vi "Configure Gamepad.vi"(6 "Cluster":T2, 7 "Configuration":T1, 8 "Slide 2":refnum<vi>, 9 "invert y":refnum<vi>, 10 "invert x":refnum<vi>, 11 "device ID":refnum<k1>) -> (3 "Configuration":T1)   [LabVIEW 2012]
uses:
  <vilib>/Utility/miscctls.llb/LVPointTypeDef.ctl
  <vilib>/Utility/inputDevices.llb/joystickAcquire.vi
  <vilib>/Utility/file.llb/Write To Spreadsheet File (I64).vi
  <vilib>/Utility/file.llb/Read From Spreadsheet File (I64).vi
panel:
  out "down":u16(ring) items=["X+", "X-", "Y+", "Y-"]
  out "left":u16(ring) items=["X+", "X-", "Y+", "Y-"]
  in  "right":u16(ring) items=["X+", "X-", "Y+", "Y-"]
  out "V":i32
  out "U":i32
  out "Left Y":i32
  out "B":i32
  out "A":i32
  out "Left X":i32
  out "Right Y":i32
  out "Right X":i32
  in  "close_button":bool
  in  "up":u16(ring) items=["X+", "X-", "Y+", "Y-"]
  in  "load":bool
  in  "save":bool
  in  "Invert":bool
  in  "Invert":bool=TRUE
  in  "Slide":cluster{u32, u32}(slide)={7, 2} scale=0.0..7.0
  out "Settings Refrences":T2
  in  "xr":u16(ring)=1 items=["1 X"=1, "2 A"=2, "3 B"=3, "4 Y"=4, "5 LB"=5, "6 RB"=6, "7 LT"=7, "8 RT"=8, "9 Back"=9]
  in  "yf":u16(ring)=4 items=["1 X"=1, "2 A"=2, "3 B"=3, "4 Y"=4, "5 LB"=5, "6 RB"=6, "7 LT"=7, "8 RT"=8, "9 Back"=9]
  in  "yr":u16(ring)=2 items=["1 X"=1, "2 A"=2, "3 B"=3, "4 Y"=4, "5 LB"=5, "6 RB"=6, "7 LT"=7, "8 RT"=8, "9 Back"=9]
  in  "xf":u16(ring)=3 items=["1 X"=1, "2 A"=2, "3 B"=3, "4 Y"=4, "5 LB"=5, "6 RB"=6, "7 LT"=7, "8 RT"=8, "9 Back"=9]
  in  "yr xr 2":u16(ring)=7 items=["1 X"=1, "2 A"=2, "3 B"=3, "4 Y"=4, "5 LB"=5, "6 RB"=6, "7 LT"=7, "8 RT"=8, "9 Back"=9]
  in  "yr xf 2":u16(ring)=8 items=["1 X"=1, "2 A"=2, "3 B"=3, "4 Y"=4, "5 LB"=5, "6 RB"=6, "7 LT"=7, "8 RT"=8, "9 Back"=9]
  in  "yf xr 2":u16(ring)=5 items=["1 X"=1, "2 A"=2, "3 B"=3, "4 Y"=4, "5 LB"=5, "6 RB"=6, "7 LT"=7, "8 RT"=8, "9 Back"=9]
  in  "yf xf 2":u16(ring)=6 items=["1 X"=1, "2 A"=2, "3 B"=3, "4 Y"=4, "5 LB"=5, "6 RB"=6, "7 LT"=7, "8 RT"=8, "9 Back"=9]
  in  "halt 2":u16(ring)=9 items=["1 X"=1, "2 A"=2, "3 B"=3, "4 Y"=4, "5 LB"=5, "6 RB"=6, "7 LT"=7, "8 RT"=8, "9 Back"=9]
  # "Control-sticks"
  # "Button mapping"
  # "Instructions\nDrag the X (green) and Y (red) MicroDrive-axis selectors to the name of a Gamepad Control-stick. \n\nNOTE: To identify your desired Control-stick, toggle the Control-stick while watching \"Readings\".\n\n."
  # "Instructions:\nClick on the text in a square to list Gamepad button options. The selected button will move the corresponding axis of the MicroDrive.\n\nThese settings effect the Gamepad buttons, and the  buttons/limit-lights of the main window."
  # "Axis"
  # "Selection"
  # "Readings"
  # "X Axis"
  # "Y Axis"
  # "CAUTION: The Gamepad's \"Mode\" button will disable the Control-sticks"
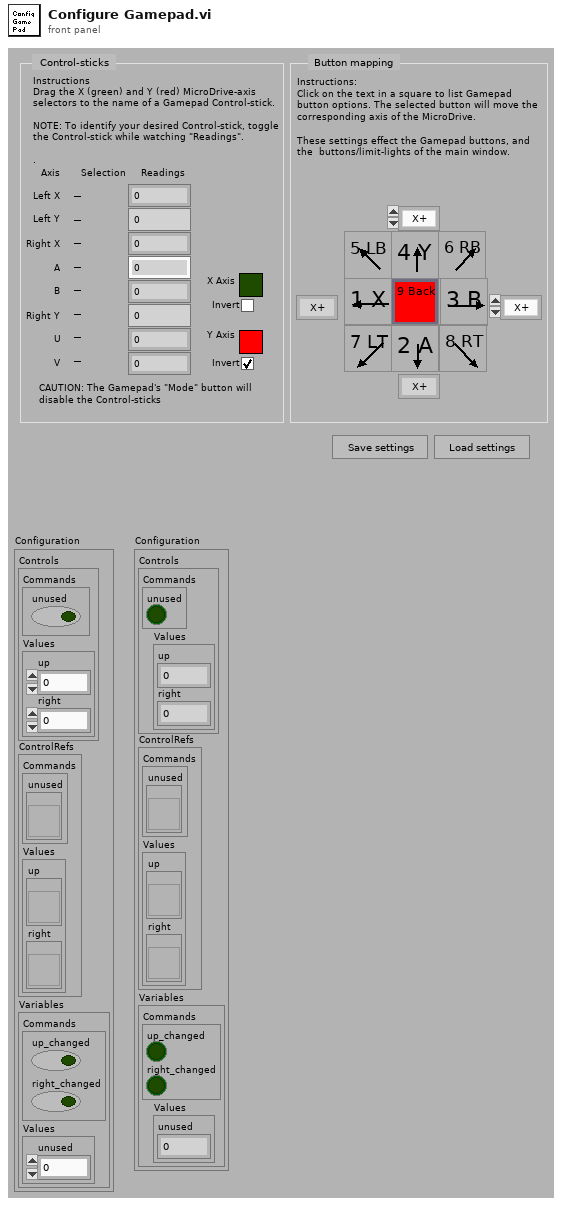
[diagram p1: front panel]
types:
  T1 = cluster{"Controls":cluster{"Commands":cluster{"unused":bool}, "Values":cluster{"up":u16, "right":u16}}, "ControlRefs":cluster{"Commands":cluster{"unused":refnum<vi>}, "Values":cluster{"up":refnum<vi>, "right":refnum<vi>}}, "Variables":cluster{"Commands":cluster{"up_changed":bool, "right_changed":bool}, "Values":cluster{"unused":i32}}}
  T2 = cluster{"xr":refnum<vi>, "yr":refnum<vi>, "xf":refnum<vi>, "yf":refnum<vi>, "yf xr 2":refnum<vi>, "yf xf 2":refnum<vi>, "yr xr 2":refnum<vi>, "yr xf 2":refnum<vi>, "halt 2":refnum<vi>}
  T3 = typedef "LVPointTypeDef.ctl" = cluster{"Horizontal":i16, "Vertical":i16}
  T4 = cluster{"X axis":i32, "Y axis":i32, "Z axis":i32, "X axis rotation":i32, "Y axis rotation":i32, "Z axis rotation":i32, "U axis":i32, "V axis":i32}
  T5 = cluster{"Right X axis":i32, "Right Y axis":i32, "Left X axis":i32, "A Axis":i32, "B Axis":i32, "Left Y axis":i32, "U axis":i32, "V axis":i32}
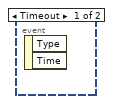
[diagram p2: hidden frame]
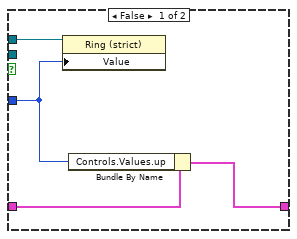
[diagram p4: hidden frame]
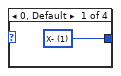
[diagram p5: hidden frame]
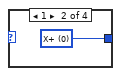
[diagram p6: hidden frame]
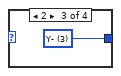
[diagram p7: hidden frame]
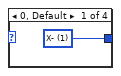
[diagram p8: hidden frame]
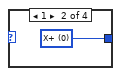
[diagram p9: hidden frame]
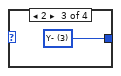
[diagram p10: hidden frame]
diagram:
  n1 = flat-sequence {
    tunnel: ["Configuration"] -> w9
    tunnel: w9 -> [w27]
    tunnel: [w26] -> w8
    tunnel: w8 -> [w29]
    tunnel: [w29] -> w22
    tunnel: [w28] -> w21
    tunnel: w22 -> [w31]
    tunnel: [w31] -> w20
    tunnel: w21 -> [w30]
    tunnel: [w35] -> w19
    tunnel: [w34] -> w18
    tunnel: w20 -> [w34]
    tunnel: [w40] -> w17
    tunnel: w19 -> [w40]
    tunnel: w18 -> [w39]
    tunnel: [w39] -> w16
    tunnel: w17 -> [w71]
    tunnel: [w71] -> w4
    tunnel: [w51] -> w2
    tunnel: w16 -> [w51]
    tunnel: w4 -> [w80]
    tunnel: [w80] -> w3
    tunnel: w2 -> [w79]
    tunnel: [w79] -> w1
    tunnel: [w82] -> w15
    tunnel: w3 -> [w82]
    tunnel: [w81] -> w14
    tunnel: w1 -> [w81]
    tunnel: w15 -> [w84]
    tunnel: [w84] -> w13
    tunnel: w14 -> [w83]
    tunnel: [w83] -> w12
    tunnel: w13 -> [w90]
    tunnel: w12 -> [w86]
    tunnel: [w88] -> w11
    tunnel: [w87] -> w10
    tunnel: w11 -> [w347]
    tunnel: w10 -> [w346]
    tunnel: [w347] -> w7
    tunnel: [w346] -> w5
    tunnel: w7 -> [w350]
    tunnel: [w350] -> w6
    tunnel: w5 -> [w349]
    tunnel: w6 -> [w351]
    frame #0 {
    }
    frame #1 {
      n2 = control-ref of="up"() -> (w25:refnum<vi>)
      n3 = control-ref of="right"() -> (w24:refnum<vi>)
      n4 = Bundle By Name(cluster=w27, "ControlRefs.Values.up"=w25, "ControlRefs.Values.right"=w24) -> (w26:T1)
    }
    frame #2 {
      n5 = control-ref of="This VI"() -> (w28:refnum<vi>)
    }
    frame #3 {
      w32 = FALSE ("Front Panel Window:Show Menu Bar")
      n6 = property class="VI"(reference=w30, "Front Panel.Minimizeable"=w32) -> ()  [unwired: 1 in, 2 out]
      n7 = property class="VI"(reference=w30, "Front Panel.ShowMenuBar"=w32) -> ()  [unwired: 1 in, 2 out]
      n8 = property class="VI"(reference=w30, "TB.Visible"=w32) -> ()  [unwired: 1 in, 2 out]
      n9 = property class="VI"(reference=w30, "Front Panel.Resizeable"=w32) -> ()  [unwired: 1 in, 2 out]
      n10 = property class="VI"(reference=w30, "Front Panel.Title"="Configure Gamepad" ("Front Panel Window:Title")) -> ()  [unwired: 1 in, 2 out]
    }
    frame #4 {
      n11 = control-ref of="This VI"() -> (w35:refnum<vi>)
      n12 = control-ref of="Pane"() -> (w36:refnum<vi>)
      n13 = property class="Pane"(reference=w36, "Origin"=T3 {"Horizontal"=0, "Vertical"=0}) -> ()  [unwired: 1 in, 2 out]
      n14 = property class="VI"(reference=w35, "GrowByDefault"=TRUE ("Expand When Dropped As SubVI")) -> ()  [unwired: 1 in, 2 out]
    }
    frame #5 {
      n15 = control-ref of="xr"() -> (w50:refnum<vi>)
      n16 = control-ref of="yr"() -> (w49:refnum<vi>)
      n17 = control-ref of="xf"() -> (w48:refnum<vi>)
      n18 = control-ref of="yf"() -> (w47:refnum<vi>)
      n19 = control-ref of="yf xr 2"() -> (w46:refnum<vi>)
      n20 = control-ref of="yf xf 2"() -> (w45:refnum<vi>)
      n21 = control-ref of="yr xr 2"() -> (w44:refnum<vi>)
      n22 = control-ref of="yr xf 2"() -> (w43:refnum<vi>)
      n23 = control-ref of="halt 2"() -> (w42:refnum<vi>)
      n24 = Bundle("xr"=w50, "yr"=w49, "xf"=w48, "yf"=w47, "yf xr 2"=w46, "yf xf 2"=w45, "yr xr 2"=w44, "yr xf 2"=w43, "halt 2"=w42) -> (→"Settings Refrences":T2)  [unwired: 1 out]
    }
    frame #6 {
      w63 = u32 7 ("x")
      n25 = local read "Settings Refrences"() -> (w57:T2)
      n26 = local read "Slide 2"() -> (w53:refnum<vi>)
      n27 = local read "Cluster"() -> (w55:T2)
      n28 = local read "invert x"() -> (w54:refnum<vi>)
      n29 = local read "invert y"() -> (w52:refnum<vi>)
      n30 = property on="Property Node" class="Slide (strict)"(reference=w53) -> ("Value"=w66:cluster{u32, u32})  [unwired: 1 in, 2 out]
      n31 = Cluster To Array(cluster=w55) -> (array=w69:refnum<vi>[])
      n32 = Cluster To Array(cluster=w57) -> (array=w70:refnum<vi>[])
      n33 = property on="Property Node" class="Bool (strict)"(reference=w52) -> ("Value"=w60:bool)  [unwired: 1 in, 2 out]
      n34 = property on="Property Node" class="Bool (strict)"(reference=w54) -> ("Value"=w68:bool)  [unwired: 1 in, 2 out]
      n35 = for {
        tunnel: w70 -> [w73] mode=indexing
        tunnel: w69 -> [w74] mode=indexing
        n36 = property on="Property Node" class="Ring (strict)"(reference=w74) -> ("Value"=w72:u16)  [unwired: 1 in, 2 out]
        n37 = property on="Property Node" class="Ring (strict)"(reference=w73, "Value"=w72) -> ()  [unwired: 1 in, 2 out]
      }
      n38 = control-ref of="invert y"() -> (w56:refnum<vi>)
      n39 = Unbundle(w66) -> (w65:u32, w64:u32)
      n40 = control-ref of="invert x"() -> (w59:refnum<vi>)
      n41 = Subtract(x=w63, y=w65) -> (x-y=w62:u32)
      n42 = Subtract(x=w63, y=w64) -> (x-y=w61:u32)
      n43 = property on="Property Node" class="Bool (strict)"(reference=w56, "Value"=w60) -> ()  [unwired: 1 in, 2 out]
      n44 = property on="Property Node" class="Bool (strict)"(reference=w59, "Value"=w68) -> ()  [unwired: 1 in, 2 out]
      n45 = control-ref of="Slide"() -> (w58:refnum<vi>)
      n46 = Bundle(w62, w61) -> (w67:cluster{u32, u32})  [unwired: 1 out]
      n47 = property on="Property Node" class="Slide (strict)"(reference=w58, "Value"=w67) -> ()  [unwired: 1 in, 2 out]
    }
    frame #7 {
      n48 = Unbundle By Name(w79) -> ("ControlRefs.Values.up"=w78:refnum<vi>, "Controls.Values.up"=w77:u16, "ControlRefs.Values.right"=w76:refnum<vi>, "Controls.Values.right"=w75:u16)
      n49 = property class="Ring (strict)"(reference=w78, "Value"=w77) -> ()  [unwired: 1 in, 2 out]
      n50 = property class="Ring (strict)"(reference=w76, "Value"=w75) -> ()  [unwired: 1 in, 2 out]
    }
    frame #8 {
    }
    frame #9 {
      n51 = property class="VI"(reference=w84, "GrowByDefault"=FALSE ("Expand When Dropped As SubVI")) -> ()  [unwired: 1 in, 2 out]
    }
    frame #10 {
      n52 = while {
        tunnel: w90 -> [w136]
        tunnel: [w95] -> w88
        shift-right: [w94] -> w87
        shift-left: w86 -> [w93]
        stop <- w135 stop-if-true
        n53 = flat-sequence {
          tunnel: w136 -> [w137]
          tunnel: w93 -> [w138]
          tunnel: [w138] -> w119
          tunnel: [w137] -> w106
          tunnel: [w148] -> w109
          tunnel: w119 -> [w147]
          tunnel: [w140] -> w107
          tunnel: w106 -> [w140]
          tunnel: w109 -> [w150]
          tunnel: [w149] -> w108
          tunnel: w107 -> [w151]
          tunnel: [w151] -> w105
          tunnel: [w189] -> w118
          tunnel: w108 -> [w189]
          tunnel: w105 -> [w188]
          tunnel: [w188] -> w103
          tunnel: ["Slide"] -> w124
          tunnel: [w205] -> w122
          tunnel: [w204] -> w120
          tunnel: w118 -> [w203]
          tunnel: [w203] -> w116
          tunnel: [w202] -> w104
          tunnel: w103 -> [w202]
          tunnel: w124 -> [w231]
          tunnel: [w231] -> w123
          tunnel: w122 -> [w230]
          tunnel: [w230] -> w121
          tunnel: w120 -> [w229]
          tunnel: [w220] -> w117
          tunnel: w116 -> [w220]
          tunnel: w104 -> [w219]
          tunnel: [w219] -> w101
          tunnel: [w238] -> w134
          tunnel: [w237] -> w133
          tunnel: w123 -> [w237]
          tunnel: [w235] -> w128
          tunnel: w121 -> [w234]
          tunnel: [w234] -> w125
          tunnel: w117 -> [w233]
          tunnel: [w233] -> w115
          tunnel: [w232] -> w102
          tunnel: w101 -> [w232]
          tunnel: w134 -> [w254]
          tunnel: [w254] -> w132
          tunnel: w133 -> [w253]
          tunnel: [w253] -> w130
          tunnel: w128 -> [w255]
          tunnel: [w255] -> w126
          tunnel: w125 -> [w248]
          tunnel: w115 -> [w244]
          tunnel: [w244] -> w114
          tunnel: w102 -> [w247]
          tunnel: [w247] -> w100
          tunnel: w132 -> [w290]
          tunnel: [w290] -> w131
          tunnel: w130 -> [w289]
          tunnel: [w289] -> w129
          tunnel: [w287] -> w127
          tunnel: w126 -> [w287]
          tunnel: w114 -> [w284]
          tunnel: [w284] -> w112
          tunnel: w100 -> [w285]
          tunnel: [w285] -> w99
          tunnel: w131 -> [_]
          tunnel: w129 -> [_]
          tunnel: w127 -> [_]
          tunnel: [w323] -> w113
          tunnel: w112 -> [w323]
          tunnel: w99 -> [w322]
          tunnel: [w322] -> w96
          tunnel: w113 -> [w328]
          tunnel: [w328] -> w110
          tunnel: [w327] -> w97
          tunnel: w96 -> [w327]
          tunnel: [w339] -> w111
          tunnel: w110 -> [w339]
          tunnel: [w338] -> w98
          tunnel: w97 -> [w338]
          tunnel: ["close_button"] -> w135
          tunnel: w111 -> [w344]
          tunnel: [w344] -> w94
          tunnel: w98 -> [w343]
          tunnel: [w343] -> w95
          frame #0 {
            n54 = property class="VI"(reference=w137, "Front Panel.IsFrontmost"=TRUE ("Front Panel Window:Is Frontmost")) -> ()  [unwired: 1 in, 2 out]
          }
          frame #1 {
            n55 = Unbundle By Name(w147) -> ("Controls.Values.up"=w144:u16, "Controls.Values.right"=w145:u16)
            n56 = Not Equal?(x="up", y=w144) -> (x != y?=w146:bool)
            n57 = Not Equal?(x=w145, y="right") -> (x != y?=w141:bool)
            n58 = Bundle By Name(cluster=w147, "Controls.Values.up"="up", "Controls.Values.right"="right", "Variables.Commands.up_changed"=w146, "Variables.Commands.right_changed"=w141) -> (w148:T1)
          }
          frame #2 {
            n59 = Unbundle By Name(w150) -> ("Controls.Values.up"=w169:u16, "Controls.Values.right"=w166:u16)
            n60 = Unbundle By Name(w150) -> ("Controls.Values.up"=w158:u16, "Controls.Values.right"=w161:u16)
            n61 = Unbundle By Name(w150) -> ("ControlRefs.Values.up"=w154:refnum<vi>, "ControlRefs.Values.right"=w153:refnum<vi>, "Variables.Commands.up_changed"=w155:bool)
            n62 = Less Or Equal?(x=w166, y=u16 1) -> (x <= y?=w164:bool)
            n63 = Greater?(x=w161, y=u16 1) -> (0:w163:bool)
            n64 = Less Or Equal?(x=w169, y=u16 1) -> (x <= y?=w165:bool)
            n65 = Greater?(x=w158, y=u16 1) -> (0:w162:bool)
            n66 = Compound Arithmetic op=AND(w165, w164) -> (w152:bool)
            n67 = Compound Arithmetic op=AND(w162, w163) -> (w157:bool)
            n68 = Compound Arithmetic op=OR(w152, w157) -> (w156:bool)
            n69 = case shown="True" w156 {
              tunnel: w155 -> [_ w179]
              tunnel: w154 -> [_ w178]
              tunnel: w153 -> [_ w177]
              tunnel: w152 -> [_ w176]
              tunnel: w150 -> [w170 w172]
              tunnel: [w170 w171] -> w149
              frame False {
              }
              frame True {
                n70 = Select(t=u16 2 ("Controls.Values.up"), s=w176, f=u16 1 ("Controls.Values.up")) -> (s? t:f=w173:u16)
                n71 = case shown="True" w179 {
                  tunnel: w178 -> [w183 _]
                  tunnel: w177 -> [_ w187]
                  tunnel: w173 -> [w180 w184]
                  tunnel: w172 -> [w182 w186]
                  tunnel: [w181 w185] -> w171
                  frame False {
                    n72 = property class="Ring (strict)"(reference=w183, "Value"=w180) -> ()  [unwired: 1 in, 2 out]
                    n73 = Bundle By Name(cluster=w182, "Controls.Values.up"=w180) -> (w181:T1)
                  }
                  frame True {
                    n74 = Bundle By Name(cluster=w186, "Controls.Values.right"=w184) -> (w185:T1)
                    n75 = property class="Ring (strict)"(reference=w187, "Value"=w184) -> ()  [unwired: 1 in, 2 out]
                  }
                }
              }
            }
          }
          frame #3 {
            n76 = Unbundle By Name(w189) -> ("Controls.Values.right"=w191:u16)
            n77 = Unbundle By Name(w189) -> ("Controls.Values.up"=w190:u16)
            n78 = case shown="3" w190 {
              tunnel: [w198 w199 w200 w201] -> w193
              frame 0, Default {
                w198 = u16 1 items=["X+", "X-", "Y+", "Y-"] ("up")
              }
              frame 1 {
                w199 = u16 0 items=["X+", "X-", "Y+", "Y-"] ("up")
              }
              frame 2 {
                w200 = u16 3 items=["X+", "X-", "Y+", "Y-"] ("up")
              }
              frame 3 {
                w201 = u16 2 items=["X+", "X-", "Y+", "Y-"] ("up")
              }
            }
            "down" <- w193
            n79 = case shown="3" w191 {
              tunnel: [w194 w195 w196 w197] -> w192
              frame 0, Default {
                w194 = u16 1 items=["X+", "X-", "Y+", "Y-"] ("up")
              }
              frame 1 {
                w195 = u16 0 items=["X+", "X-", "Y+", "Y-"] ("up")
              }
              frame 2 {
                w196 = u16 3 items=["X+", "X-", "Y+", "Y-"] ("up")
              }
              frame 3 {
                w197 = u16 2 items=["X+", "X-", "Y+", "Y-"] ("up")
              }
            }
            "left" <- w192
          }
          frame #4 {
            w215 = u32 7 ("x")
            n80 = Unbundle("Slide") -> (w213:u32, w214:u32)
            n81 = Subtract(x=w215, y=w213) -> (x-y=w216:u32)
            n82 = Subtract(x=w215, y=w214) -> (x-y=w217:u32)
            n83 = call-poly <vilib>:"Acquire Input Data.vi"("device ID"="device ID") -> ("axis info"=w211:T4)  [unwired: 1 in, 17 out]
            n84 = Bundle(cluster="Slide", w216, w217) -> (w218:cluster{u32, u32})
            n85 = call "invert joystick cluster values.vi"("Invert Y"="Invert", "Invert X"="Invert", "Slide"=w218, "Joystick Readings"=w211) -> ("Joystick Readings 2"=w204:T5)  [unwired: 7 out]
            n86 = Boolean To (0,1)(Boolean="Invert") -> (0, 1=w207:i16)
            n87 = Boolean To (0,1)(Boolean="Invert") -> (0, 1=w206:i16)
            n88 = Build Array(w207, w206) -> (w205:i16[])
          }
          frame #5 {
            n89 = Unbundle By Name(w229) -> ("Right X axis"=→"Left X":i32, "Right Y axis"=→"Left Y":i32, "Left X axis"=→"Right X":i32, "A Axis"=→"A":i32, "B Axis"=→"B":i32, "Left Y axis"=→"Right Y":i32, "U axis"=→"U":i32, "V axis"=→"V":i32)
          }
          frame #6 {
            n90 = local read "Settings Refrences"() -> (w240:T2)
            n91 = Cluster To Array(cluster=w240) -> (array=w235:refnum<vi>[])
            n92 = Cluster To Array(cluster="Cluster") -> (array=w236:refnum<vi>[])
            n93 = for {
              tunnel: w236 -> [w242] mode=indexing
              tunnel: w235 -> [w243] mode=indexing
              tunnel: [w241] -> w238 mode=indexing
              n94 = property on="Property Node" class="Ring (strict)"(reference=w243) -> ("Value"=w241:u16)  [unwired: 1 in, 2 out]
              n95 = property on="Property Node" class="Ring (strict)"(reference=w242, "Value"=w241) -> ()  [unwired: 1 in, 2 out]
            }
          }
          frame #7 {
            n96 = Unbundle By Name(w244) -> ("Controls.Values.up"=w246:u16, "Controls.Values.right"=w245:u16)
            n97 = Unbundle(w253) -> (w252:u32, w251:u32)
            n98 = Build Array (concatenate)(w254, w252, w251, w248, w246, w245) -> (w250:u32[])
            n99 = case shown="True" "save" {
              tunnel: w250 -> [_ w271]
              frame False {
              }
              frame True {
                n100 = Get Date/Time String() -> (date string=w259:string, time string=w268:string)  [unwired: 3 out]
                n101 = call <vilib>:"Space Constant.vi"() -> ("String"=w267:string)
                n102 = Concatenate Strings(w259, w267, w268) -> (w260:string)
                n103 = control-ref of="This Application"() -> (w275:refnum<vi>)
                n104 = Search and Replace String(replace all?=TRUE ("replace all? (F)"), input string=w260, search string=":") -> (result string=w262:string)  [unwired: 1 in, 7 out]
                n105 = Search and Replace String(replace all?=TRUE ("replace all? (F)"), input string=w262, search string="/", replace string="-" ("replace string (\"\")")) -> (result string=w258:string)  [unwired: 1 in, 6 out]
                n106 = property class="App"(reference=w275) -> ("App.Dir"=w277:path)  [unwired: 1 in, 2 out]
                n107 = Concatenate Strings("gamepad  " ("string"), w258) -> (w256:string)
                n108 = call "File Dialog"("default name"=w256, "pattern (all files)"="*.txt") -> ("selected path"=w273:path, "cancelled"=w272:bool, "error out"=w269:errorcluster)  [unwired: 5 in, 6 out]
                n109 = Build Path(base path=w277, name or relative path="config.txt") -> (appended path=w274:path)
                n110 = case shown="False" w272 {
                  tunnel: w274 -> [w283 _]
                  tunnel: w273 -> [w279 _]
                  tunnel: w271 -> [w278 _]
                  tunnel: w269 -> [_ _]
                  frame False {
                    n111 = call-poly <vilib>:"Write To Spreadsheet File.vi"("transpose? (no:F)"=TRUE, "1D data"=w278, "file path (dialog if empty)"=w279) -> ("new file path (Not A Path if cancelled)"=w282:path)  [unwired: 3 in, 2 out]
                    n112 = Path To String(path=w282) -> (string=w280:string)
                    n113 = Write to Text File(file (use dialog)=w283, text=w280) -> ()  [unwired: 1 in, 4 out]
                  }
                  frame True {
                  }
                }
              }
            }
          }
          frame #8 {
            n114 = control-ref of="Slide"() -> (w286:refnum<vi>)
            n115 = case shown="True" "load" {
              tunnel: w287 -> [_ w296]
              tunnel: w286 -> [_ w297]
              tunnel: w284 -> [_ w291]
              frame False {
              }
              frame True {
                n116 = call "File Dialog2"("pattern (all files)"="*.txt") -> ("selected path"=w294:path, "cancelled"=w292:bool, "error out"=w293:errorcluster)  [unwired: 6 in, 6 out]
                n117 = case shown="False" w292 {
                  tunnel: w297 -> [w315 _]
                  tunnel: w296 -> [w313 _]
                  tunnel: w294 -> [w303 _]
                  tunnel: w293 -> [_ _]
                  tunnel: w291 -> [w299 _]
                  frame False {
                    n118 = call-poly <vilib>:"Read From Spreadsheet File.vi"("transpose (no:F)"=TRUE ("transpose? (no:F)"), "file path (dialog if empty)"=w303) -> ("first row"=w304:i64[])  [unwired: 2 in, 7 out]
                    n119 = Array Size(array=w313) -> (size(s)=w319:i32)
                    n120 = Split 1D Array(array=w304, index=w319) -> (first subarray=w312:i64[], second subarray=w318:i64[])
                    n121 = Index Array(array=w318) -> (element #1=w316:i64, element #2=w317:i64, element #3=w309:i64, element #4=w306:i64, element #5=w301:i64, element #6=w298:i64)  [unwired: 6 in]
                    n122 = Bundle(w316, w317) -> (w314:cluster{i64, i64})  [unwired: 1 out]
                    n123 = property class="Slide (strict)"(reference=w315, "Value"=w314) -> ()  [unwired: 1 in, 2 out]
                    n124 = control-ref of="Invert"() -> (w311:refnum<vi>)
                    n125 = Greater Than 0?(x=w309) -> (x > 0?=w308:bool)
                    n126 = property class="Bool (strict)"(reference=w311, "Value"=w308) -> ()  [unwired: 1 in, 2 out]
                    n127 = control-ref of="Invert"() -> (w310:refnum<vi>)
                    n128 = Greater Than 0?(x=w306) -> (x > 0?=w307:bool)
                    n129 = property class="Bool (strict)"(reference=w310, "Value"=w307) -> ()  [unwired: 1 in, 2 out]
                    n130 = Unbundle By Name(w299) -> ("ControlRefs.Values.up"=w302:refnum<vi>)
                    n131 = property class="Ring (strict)"(reference=w302, "Value"=w301) -> ()  [unwired: 1 in, 2 out]
                    n132 = Unbundle By Name(w299) -> ("ControlRefs.Values.right"=w300:refnum<vi>)
                    n133 = property class="Ring (strict)"(reference=w300, "Value"=w298) -> ()  [unwired: 1 in, 2 out]
                    n134 = for {
                      tunnel: w313 -> [w321] mode=indexing
                      tunnel: w312 -> [w320] mode=indexing
                      n135 = property class="Ring (strict)"(reference=w321, "Value"=w320) -> ()  [unwired: 1 in, 2 out]
                    }
                  }
                  frame True {
                  }
                }
              }
            }
          }
          frame #9 {
            n136 = control-ref of="invert x"() -> (w325:refnum<vi>)
            n137 = property on="Property Node" class="Bool (strict)"(reference=w325) -> ("Value"=w324:bool)  [unwired: 1 in, 2 out]
            n138 = property on="Property Node" class="Bool (strict)"(reference="invert x", "Value"=w324) -> ()  [unwired: 1 in, 2 out]
          }
          frame #10 {
            w333 = u32 7 ("x")
            n139 = control-ref of="Slide"() -> (w329:refnum<vi>)
            n140 = property on="Property Node" class="Slide (strict)"(reference=w329) -> ("Value"=w336:cluster{u32, u32})  [unwired: 1 in, 2 out]
            n141 = Unbundle(w336) -> (w335:u32, w334:u32)
            n142 = Subtract(x=w333, y=w335) -> (x-y=w332:u32)
            n143 = Subtract(x=w333, y=w334) -> (x-y=w331:u32)
            n144 = Bundle(w332, w331) -> (w337:cluster{u32, u32})  [unwired: 1 out]
            n145 = property on="Property Node" class="Slide (strict)"(reference="Slide 2", "Value"=w337) -> ()  [unwired: 1 in, 2 out]
          }
          frame #11 {
            n146 = control-ref of="invert y"() -> (w341:refnum<vi>)
            n147 = property on="Property Node" class="Bool (strict)"(reference=w341) -> ("Value"=w340:bool)  [unwired: 1 in, 2 out]
            n148 = property on="Property Node" class="Bool (strict)"(reference="invert y", "Value"=w340) -> ()  [unwired: 1 in, 2 out]
          }
          frame #12 {
          }
        }
      }
      n149 = event shown="[1] Panel Close?" {
        selector: _ -> [_ _]
        dyn-events: _ -> [_ _]
        timeout: -1 -> [_ _]
        event Timeout {
          n150 = event-data() -> ()  [unwired: 3 out]
        }
        event Panel Close? {
          n151 = event-data() -> ()  [unwired: 4 out]
          n152 = local write "close_button"(TRUE ("closed?")) -> ()
          n153 = event-data("Discard?"=TRUE) -> ()  [unwired: 1 in, 1 out]
        }
      }
    }
    frame #11 {
      w348 = FALSE  # close_button
      n154 = local write "close_button"(w348) -> ()
    }
    frame #12 {
      "Configuration" <- w349
    }
    frame #13 {
      n155 = invoke class="VI" method="FP.Close"(reference=w351) -> ()  [unwired: 2 in, 3 out]
    }
  }
